vi "configure 8 or 12kHz 5 ch resonance PXI.vi"(6 "x resonant zoom voltage":dbl, 8 "error in":errorcluster, 9 "y-voltage":dbl=2.0, 10 "Start Delay (Ticks)":i16, 11 "lines (2pi) per frame":i32=100) -> (0 "error out":errorcluster, 1 "pixels per frame":dbl, 2 "FPGA VI Reference Out":refnum<k20>, 3 "AO task out":refnum<k21>, 4 "Actual Depth 3":u32)   [LabVIEW 2012]
uses:
  <vilib>/userDefined/High Color/nirio_resource_hc.ctl
  <vilib>/DAQmx/write.llb/DAQmx Write (Analog 2D DBL NChan NSamp).vi
  GFG/GFGbooleanGet.vi
  <vilib>/FPGAPlugInAG/PXIe-7962R/niLvFpga_Open_PXIe-7962R.vi
  <vilib>/FPGAPlugInAG/PXIe-7962R/niLvFpga_Abort_PXIe-7962R.vi
  <vilib>/Utility/error.llb/Error Cluster From Error Code.vi
  <vilib>/rvi/errors/niLvFpgaAdjustHostInterfaceError.vi
  <vilib>/FPGAPlugInAG/PXIe-7962R/niLvFpga_Run_PXIe-7962R.vi
  <vilib>/DAQmx/create/channels.llb/DAQmx Create Channel (AO-Voltage-Basic).vi
  <vilib>/DAQmx/configure/timing.llb/DAQmx Timing (Sample Clock).vi
  <vilib>/DAQmx/configure/trigger.llb/DAQmx Start Trigger (Digital Edge).vi
  GFG/GFGnumericGet.vi
  GFG/GFGfpRefGet.vi
  <vilib>/DAQmx/miscellaneous.llb/DAQmx Fill In Error Info.vi
  <vilib>/rvi/interface/nirviOpenFPGA/nirviOpenFPGA.xnode
  FPGA/FPGA lvproj/FPGA Bitfiles/4chresonancescan_PXIe-7962R_5ch8or12kHzreson_D7lwWdudtb8.lvbitx
  <vilib>/rvi/interface/nirviMethod/nirviMethod.xnode
  <vilib>/rvi/interface/nirviReadWriteControl/nirviReadWriteControl.xnode
  <vilib>/rvi/errors/niLvFpgaMergeErrorWithErrorCode.vi
  GFG/GFG library.lvlib
  <vilib>/FPGAPlugInAG/PXIe-7962R/niLvFpga_ConfigureFifo_PXIe-7962R.vi
  <vilib>/FPGAPlugInAG/PXIe-7962R/niLvFpga_ReadFifo_PXIe-7962R.vi
  NiFpgaLv.dll
panel:
  out "Actual Depth 2":u32
  out "Waveform Graph":dbl[][](graph)
  in  "Requested Depth":u32=100000000
  in  "RIO Device":T1="RIO0"
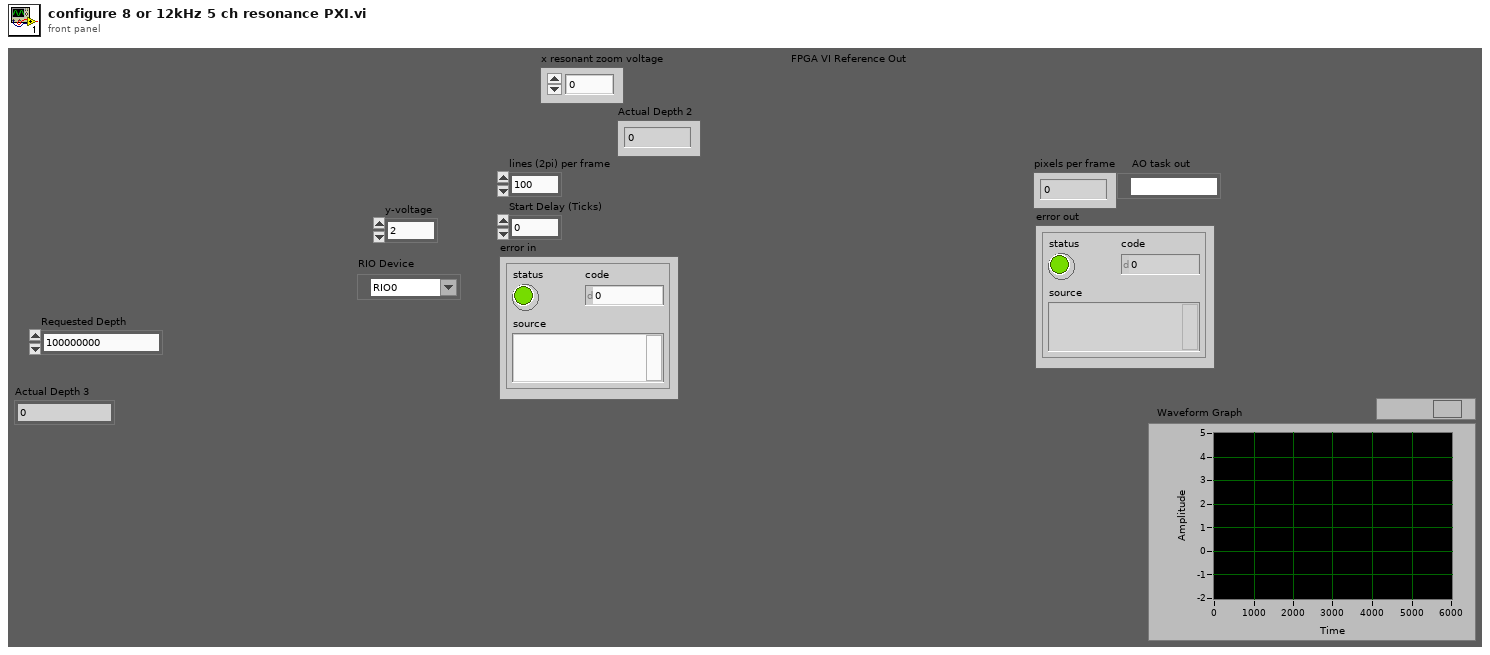
[diagram p1: front panel]
types:
  T1 = typedef "nirio_resource_hc.ctl" = tag
  T2 = enum8{"Enabled", "Disabled", "Disabled and Grayed Out"}
  T3 = cluster{"WaveformChartRef":refnum<vi>, "DigitalRef":refnum<vi>, "ArrayRef":refnum<vi>, "TabControlRef":refnum<vi>, "EnumRef":refnum<vi>, "RingRef":refnum<vi>, "BooleanRef":refnum<vi>, "KnobRef":refnum<vi>, "SlideRef":refnum<vi>, "PathRef":refnum<vi>, "StringRef":refnum<vi>, "ComboBox":refnum<vi>, "WaveformGraphRef":refnum<vi>}
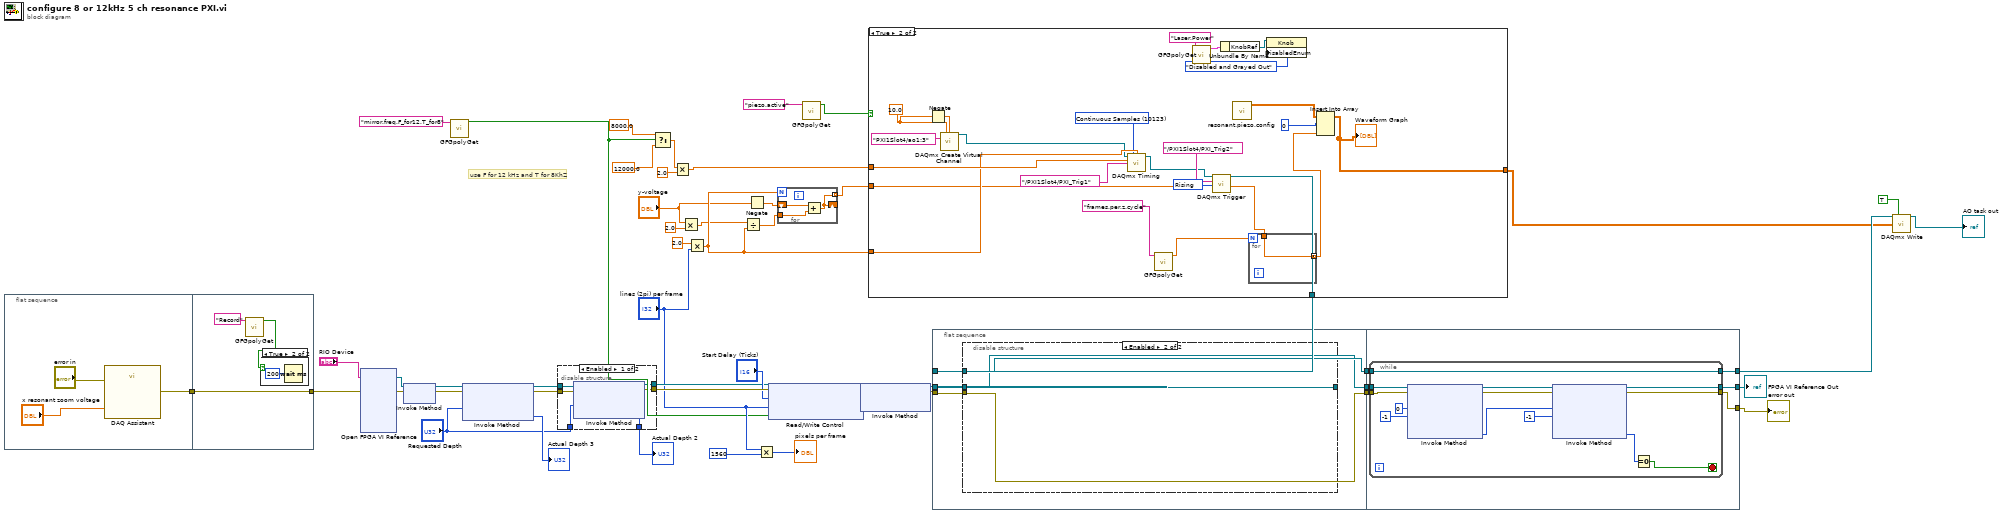
[diagram p0: block diagram]
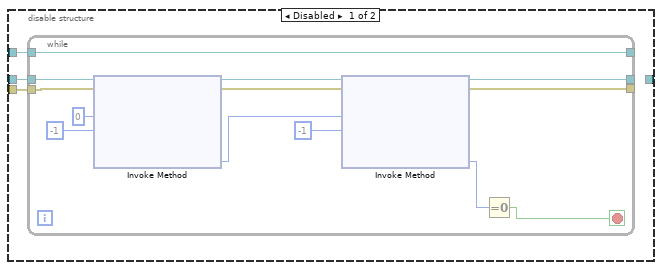
[diagram p3: hidden frame]
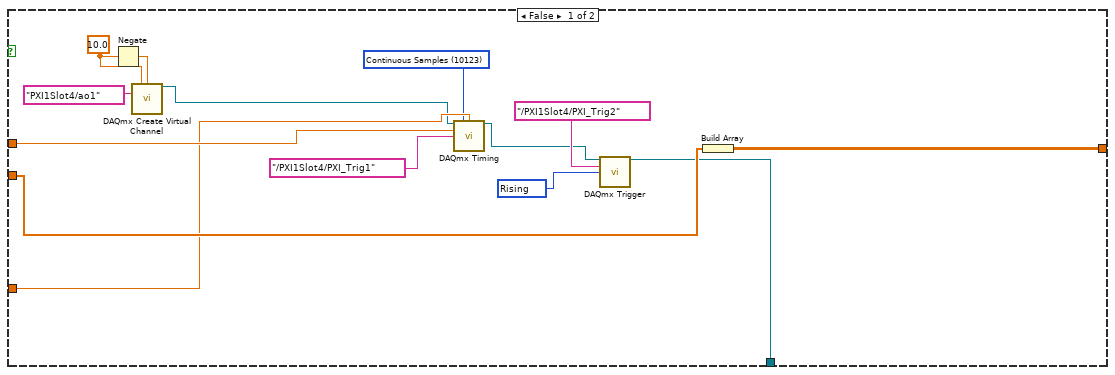
[diagram p5: hidden frame]
diagram:
  # "use F for 12 kHz and T for 8KhZ"
  n1 = flat-sequence {
    tunnel: [w50] -> w17
    tunnel: [w55] -> w25
    tunnel: w17 -> [w55]
    frame #0 {
      n2 = call "DAQ Assistant"("data"="x resonant zoom voltage", "error in"="error in") -> ("error out"=w50:errorcluster)  [unwired: 16 in, 1 out]
    }
    frame #1 {
      n3 = call-poly "GFGpolyGet.vi"("Variable Name in"="Record") -> ("Boolean"=w53:bool)  [unwired: 10 in]
      n4 = case shown="True" w53 {
        frame False {
        }
        frame True {
          n5 = Wait (ms)(milliseconds to wait=u32 200) -> ()  [unwired: 1 out]
        }
      }
    }
  }
  n6 = xnode "Open FPGA VI Reference"("error in"=w25, "resource name"="RIO Device") -> ("FPGA VI Reference Out"=w47:refnum<k20>, "error out"=w48:errorcluster)
  n7 = xnode "Invoke Method"("FPGA VI Reference In"=w47, "error in"=w48) -> ("FPGA VI Reference Out"=w10:refnum<k20>, "error out"=w11:errorcluster)
  n8 = call-poly "GFGpolyGet.vi"("Variable Name in"="mirror.freq.F_for12.T_for8") -> ("Boolean"=w2:bool)  [unwired: 10 in]
  n9 = xnode "Invoke Method"("FPGA VI Reference In"=w10, "error in"=w11, "Requested Depth"="Requested Depth") -> ("FPGA VI Reference Out"=w20:refnum<k20>, "error out"=w19:errorcluster, "Actual Depth"=→"Actual Depth 3":u32)
  n10 = disable-structure shown="Enabled" {
    disable-tunnel: [w62 w63] -> w44
    disable-tunnel: w20 -> [w61 w64]
    disable-tunnel: w19 -> [w60 w63]
    disable-tunnel: [w59 _] -> w16
    disable-tunnel: "Requested Depth" -> [w58 _]
    disable-tunnel: [w57 w64] -> w14
    frame Enabled {
      n11 = xnode "Invoke Method"("FPGA VI Reference In"=w61, "error in"=w60, "Requested Depth"=w58) -> ("FPGA VI Reference Out"=w57:refnum<k20>, "error out"=w62:errorcluster, "Actual Depth"=w59:u32)
    }
    frame Disabled {
    }
  }
  "Actual Depth 2" <- w16
  n12 = Select(t=8000.0 ("rate"), s=w2, f=12000.0 ("rate")) -> (s? t:f=w7:dbl)
  n13 = Multiply(x=w7, y=2.0) -> (x*y=w37:dbl)
  n14 = Multiply(x="y-voltage", y=2.0) -> (x*y=w32:dbl)
  n15 = Multiply(x=2.0, y="lines (2pi) per frame") -> (x*y=w36:dbl)
  n16 = Divide(x=w32, y=w36) -> (x/y=w28:dbl)
  n17 = Negate(x="y-voltage") -> (-x=w29:dbl)
  n18 = Multiply(x="lines (2pi) per frame", y=i16 1560 ("samples per period")) -> (x*y=→"pixels per frame":i32)
  n19 = xnode "Read/Write Control"("FPGA VI Reference In"=w14, "error in"=w44, "Start Delay (Ticks)"="Start Delay (Ticks)", "lines at once"="lines (2pi) per frame", "frequency (T:8kHz F:12kHz)"=w2) -> ("FPGA VI Reference Out"=w46:refnum<k20>, "error out"=w45:errorcluster)
  n20 = for {
    N: w36 -> [_]
    tunnel: w28 -> [w66]
    shift-right: [w65] -> _
    shift-left: w29 -> [w67]
    tunnel: [w65] -> w39 mode=indexing
    n21 = Add(x=w67, y=w66) -> (x+y=w65:dbl)
  }
  n22 = call-poly "GFGpolyGet.vi"("Variable Name in"="piezo.active") -> ("Boolean"=w22:bool)  [unwired: 10 in]
  n23 = xnode "Invoke Method"("FPGA VI Reference In"=w46, "error in"=w45) -> ("FPGA VI Reference Out"=w41:refnum<k20>, "error out"=w40:errorcluster)  [unwired: 1 in]
  n24 = case shown="True" w22 {
    tunnel: w39 -> [w81 w88]
    tunnel: w37 -> [w79 w103]
    tunnel: w36 -> [w76 w100]
    tunnel: [w70 w94] -> w27
    tunnel: [w68 w90] -> w24
    frame False {
      w80 = 10280 items=["Rising"=10280, "Falling"=10171] ("edge")
      w73 = 10123 items=["Finite Samples"=10178, "Continuous Samples"=10123, "Hardware Timed Single Point"=12522] ("sample mode")
      w74 = 10.0 ("maximum value")
      n25 = Negate(x=w74) -> (-x=w75:dbl)
      n26 = call-poly <vilib>:"DAQmx Create Virtual Channel.vi"("maximum value"=w74, "minimum value"=w75, "physical channels"=tag "PXI1Slot4/ao1") -> ("task out"=w71:refnum<k21>)  [unwired: 11 in, 1 out]
      n27 = call-poly <vilib>:"DAQmx Timing.vi"("task/channels in"=w71, "sample mode"=w73, "samples per channel"=w76, "rate"=w79, "source"=tag "/PXI1Slot4/PXI_Trig1") -> ("task out"=w69:refnum<k21>)  [unwired: 9 in, 1 out]
      n28 = call-poly <vilib>:"DAQmx Trigger.vi"("task/channels in"=w69, "source"=tag "/PXI1Slot4/PXI_Trig2", "edge"=w80) -> ("task out"=w70:refnum<k21>)  [unwired: 11 in, 1 out]
      n29 = Build Array(w81) -> (w68:dbl[][])
    }
    frame True {
      w104 = 10280 items=["Rising"=10280, "Falling"=10171] ("edge")
      w97 = 10123 items=["Finite Samples"=10178, "Continuous Samples"=10123, "Hardware Timed Single Point"=12522] ("sample mode")
      w98 = 10.0 ("maximum value")
      n30 = Negate(x=w98) -> (-x=w99:dbl)
      n31 = call-poly <vilib>:"DAQmx Create Virtual Channel.vi"("maximum value"=w98, "minimum value"=w99, "physical channels"=tag "PXI1Slot4/ao1:3") -> ("task out"=w95:refnum<k21>)  [unwired: 11 in, 1 out]
      n32 = call-poly <vilib>:"DAQmx Timing.vi"("task/channels in"=w95, "sample mode"=w97, "samples per channel"=w100, "rate"=w103, "source"=tag "/PXI1Slot4/PXI_Trig1") -> ("task out"=w93:refnum<k21>)  [unwired: 9 in, 1 out]
      n33 = call-poly "GFGpolyGet.vi"("Variable Name in"="frames.per.z.cycle" ("Tag in")) -> ("Numeric"=w87:dbl)  [unwired: 9 in, 1 out]
      n34 = call-poly "GFGpolyGet.vi"("Variable Name in"="Laser.Power") -> ("output cluster"=w85:T3)  [unwired: 9 in, 1 out]
      n35 = call-poly <vilib>:"DAQmx Trigger.vi"("task/channels in"=w93, "source"=tag "/PXI1Slot4/PXI_Trig2", "edge"=w104) -> ("task out"=w94:refnum<k21>)  [unwired: 11 in, 1 out]
      n36 = Unbundle By Name(w85) -> ("KnobRef"=w82:refnum<vi>)
      n37 = call "resonant.piezo.config.vi"() -> ("appended array"=w92:dbl[][])  [unwired: 11 in]
      n38 = for {
        N: w87 -> [_]
        tunnel: w88 -> [w105]
        tunnel: [w105] -> w86 mode=concatenating
      }
      n39 = property class="Knob"(reference=w82, "DisabledEnum"=T2."Disabled and Grayed Out" ("Disabled")) -> ()  [unwired: 1 in, 2 out]
      n40 = Insert Into Array(array=w92, index (row)=0 ("disabled index (col)"), new element=w86) -> (w90:dbl[][])  [unwired: 1 in]
      "Waveform Graph" <- w90
    }
  }
  n41 = flat-sequence {
    tunnel: w41 -> [w106]
    tunnel: [w106] -> w6
    tunnel: w40 -> [w108]
    tunnel: [w108] -> w5
    tunnel: w27 -> [w107]
    tunnel: [w107] -> w4
    tunnel: w6 -> [w131]
    tunnel: w5 -> [w130]
    tunnel: w4 -> [w129]
    tunnel: [w128] -> w26
    tunnel: [w126] -> w18
    tunnel: [w127] -> w1
    frame #0 {
      n42 = disable-structure shown="Enabled" {
        disable-tunnel: w106 -> [w111 w125]
        disable-tunnel: w108 -> [w110 _]
        disable-tunnel: w107 -> [w109 _]
        disable-tunnel: [_ w125] -> _
        frame Disabled {
          n43 = while {
            tunnel: w111 -> [w124]
            tunnel: w110 -> [w118]
            tunnel: [w116] -> _
            tunnel: [w115] -> _
            tunnel: w109 -> [w114]
            tunnel: [w114] -> _
            stop <- w119 stop-if-true
            n44 = xnode "Invoke Method"("FPGA VI Reference In"=w124, "error in"=w118, "Number of Elements"=u32 0, "Timeout (ms)"=-1) -> ("FPGA VI Reference Out"=w120:refnum<k20>, "error out"=w117:errorcluster, "Elements Remaining"=w113:u32)  [unwired: 1 out]
            n45 = xnode "Invoke Method"("FPGA VI Reference In"=w120, "error in"=w117, "Number of Elements"=w113, "Timeout (ms)"=-1) -> ("FPGA VI Reference Out"=w116:refnum<k20>, "error out"=w115:errorcluster, "Elements Remaining"=w112:u32)  [unwired: 1 out]
            n46 = Equal To 0?(x=w112) -> (x = 0?=w119:bool)
          }
        }
        frame Enabled {
        }
      }
    }
    frame #1 {
      n47 = while {
        tunnel: w131 -> [w144]
        tunnel: w130 -> [w136]
        tunnel: [w134] -> w127
        tunnel: [w133] -> w126
        tunnel: w129 -> [w132]
        tunnel: [w132] -> w128
        stop <- w137 stop-if-true
        n48 = xnode "Invoke Method"("FPGA VI Reference In"=w144, "error in"=w136, "Number of Elements"=u32 0, "Timeout (ms)"=-1) -> ("FPGA VI Reference Out"=w140:refnum<k20>, "error out"=w135:errorcluster, "Elements Remaining"=w139:u32)  [unwired: 1 out]
        n49 = xnode "Invoke Method"("FPGA VI Reference In"=w140, "error in"=w135, "Number of Elements"=w139, "Timeout (ms)"=-1) -> ("FPGA VI Reference Out"=w134:refnum<k20>, "error out"=w133:errorcluster, "Elements Remaining"=w138:u32)  [unwired: 1 out]
        n50 = Equal To 0?(x=w138) -> (x = 0?=w137:bool)
      }
    }
  }
  n51 = call-poly <vilib>:"DAQmx Write.vi"("task/channels in"=w26, "auto start"=TRUE, "data"=w24) -> ("task out"=→"AO task out":refnum<k21>)  [unwired: 10 in, 2 out]
  "error out" <- w18
  "FPGA VI Reference Out" <- w1
